vi "GetFileData.vi"(7 "LabVIEW Web Service Request":refnum<class "Web Request.lvclass">, 10 "FileName":string) -> ()   [LabVIEW 2019]
uses:
  <vilib>/wsapi/Web Request.lvclass
  IndoorData_class/IndoorData.lvclass
panel:
  # "Use the Web Service Request input terminal to call the VIs on the Web Services palette. Do not remove it from the connector pane unless you don't need access to the palette."
  # "Each additional control wired to the connector pane will be available as an input in the URL. To include an indicator in terminal-mode output (the default setting), it must also be wired to the connector pane."
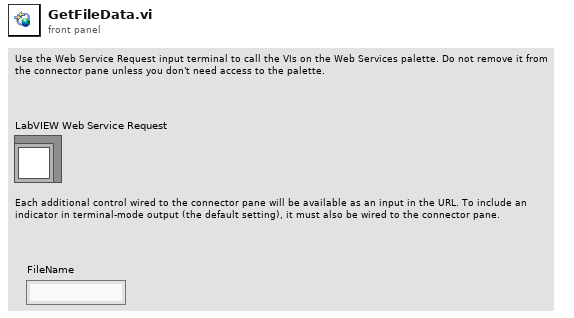
[diagram p1: front panel]
types:
  T1 = typedef "IndoorData.lvclass/BufferedReadings.ctl" = cluster{"Time":dbl[], "Temp":dbl[], "RH":dbl[]}
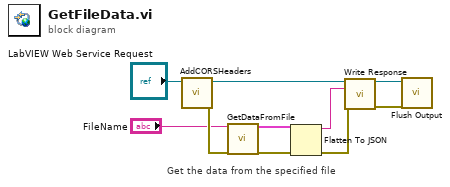
[diagram p0: block diagram]
diagram:
  # "Get the data from the specified file"
  n1 = call "AddCORSHeaders.vi"("LabVIEW Web Service Request"="LabVIEW Web Service Request") -> ("error out"=w8:errorcluster, "LabVIEW Web Service Request out"=w7:refnum<class "Web Request.lvclass">)  [unwired: 9 in]
  n2 = call "GetDataFromFile.vi"("FileName"="FileName", "error in (no error)"=w8) -> ("FileData"=w1:T1, "error out"=w6:errorcluster)  [unwired: 15 in, 1 out]
  n3 = Flatten To JSON(anything=w1, error in (no error)=w6) -> (JSON string=w5:string, 11:w4:errorcluster)  [unwired: 1 in]
  n4 = call <vilib>:"Write Response.vi"("LabVIEW Web Service Request"=w7, "response string"=w5, "error in (no error)"=w4) -> ("LabVIEW Web Service Request out"=w10:refnum<class "Web Request.lvclass">, "error out"=w9:errorcluster)  [unwired: 11 in]
  n5 = call <vilib>:"Flush Output.vi"("LabVIEW Web Service Request"=w10, "error in (no error)"=w9) -> ()  [unwired: 12 in, 2 out]
